vi "Configuration.vi"(8 "error in (no error)":errorcluster, 10 "RoiFilter":T1, 11 "Sensor in":refnum<class "Sensor.lvclass">) -> (0 "error out":errorcluster, 3 "Sensor out":refnum<class "Sensor.lvclass">)   [LabVIEW 2018, in "Sensor.lvlib" / "Sensor.lvclass"]
uses:
  Sensor.lvclass
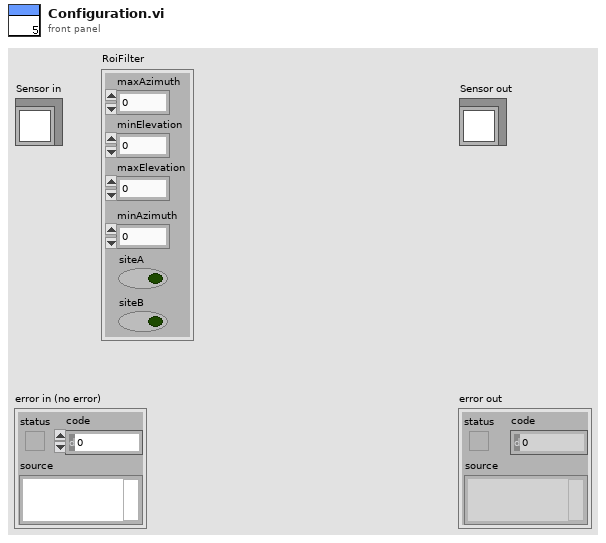
[diagram p1: front panel]
types:
  T1 = cluster{"minAzimuth":dbl, "maxAzimuth":dbl, "minElevation":dbl, "maxElevation":dbl, "siteA":bool, "siteB":bool}
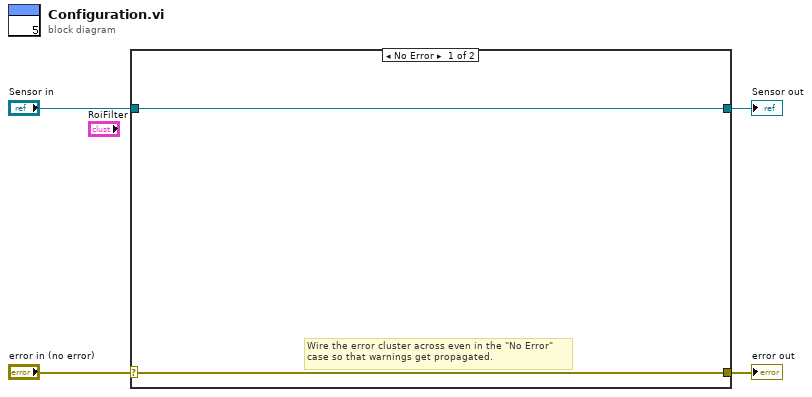
[diagram p0: block diagram]
diagram:
  n1 = case shown="No Error" "error in (no error)" {
    selector: "error in (no error)" -> [w5 w8]
    tunnel: [w5 w8] -> w3
    tunnel: [w6 w7] -> w1
    tunnel: "Sensor in" -> [w6 w7]
    frame No Error {
      # "Wire the error cluster across even in the \"No Error\"\ncase so that warnings get propagated."
    }
    frame Error {
    }
  }
  "error out" <- w3
  "Sensor out" <- w1
